vi "PCO_RecorderCreate.vi"(1 "wRecMode":u16(ring)=2 items=["PCO_RECORDER_MODE_FILE"=1, "PCO_RECORDER_MODE_MEMORY"=2, "PCO_RECORDER_MODE_CAMRAM"=3], 5 "phCamArr":u64[](array[numeric])=array[4097 elements], 7 "dwImgDistributionArr":u32[](array[numeric]), 9 "szDrive":path, 11 "error in (no error)":errorcluster {"code" format="%x"}, 12 "wFlags":u16 format="%04x") -> (4 "phRec out":u64, 6 "ErrorMessage":i32 format="%x", 8 "dwMaxImgCountArr":u32[](array[numeric]), 15 "error out":errorcluster {"code" format="%x"})   [LabVIEW 2019, in "Recorder.lvlib"]
doc: "<b>Description:</b>\nThis function creates the one and only instance of the recorder. It takes an array of handles to the required cameras as input parameter. If the function succeeds, those handles may not be used outside of the recorder until PCO_RecorderDelete is called. The main task of this function is to calculate the maximum recordable number of images for every camera by checking the available memory (RAM or Disk depending on the recorder mode) and the required distribution of the memory to the single cameras (e.g camera 1 should get twice as much available memory as camera 2, than the distribution would be [2, 1]). If the recorder is used in record to file mode, also the drive and the file type have to be specified, otherwise those parameters are just ignored.\nFunction will be rejected with error if a recorder was already created.\n\n<b>Note: </b>For file mode this function returns a warning, if the file name of the specified path already exists.\nThe function will be rejected with error if a recorder was already created.\n\n<b>Supported camera type:</b>\nAll cameras"
uses:
  Recorder.lvlib
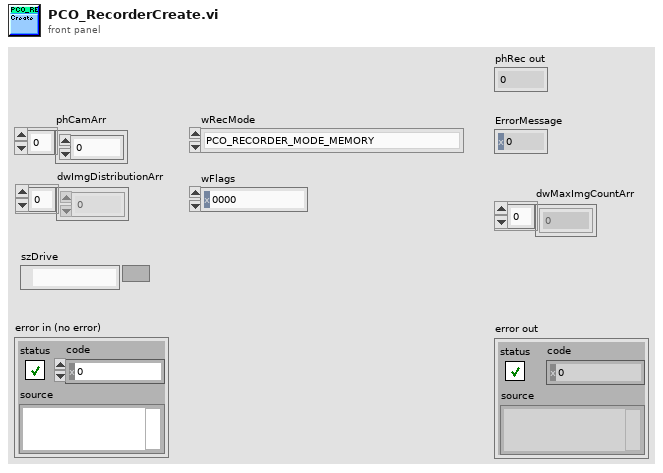
[diagram p1: front panel]
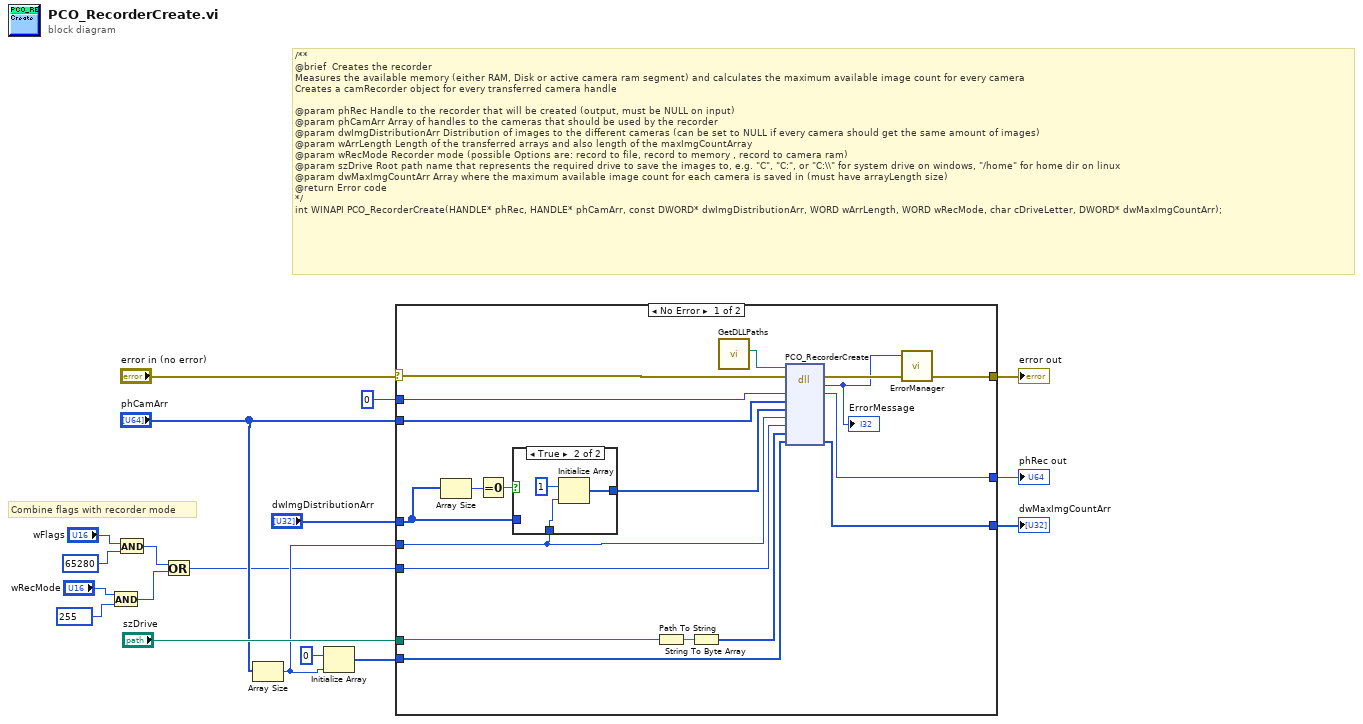
[diagram p0: block diagram]
diagram:
  # "Combine flags with recorder mode"
  # "/**\n@brief \tCreates the recorder\nMeasures the available memory (either RAM, Disk or active camera ram segment) and calculates the maximum available image count for every camera\nCreates a camRecorder object for every transferred camera handle\n\n@param phRec Handle to the recorder that will be created (output, must be NULL on input)\n@param phCamArr Array of handles to the cameras that should be used by the recorder\n@param dwImgDistributionArr Distribution of images to the different cameras (can be set to NULL if every camera should get the same amount of images)\n@param wArrLength Length of the transferred arrays and also length of the maxImgCountArray\n@param wRecMode Recorder mode (possible Options are: record to file, record to memory , record to camera ram)\n@param szDrive Root path name that represents the required drive to save the images to, e.g. \"C\", \"C:\", or \"C:\\\\\" for system drive on windows, \"/home\" for home dir on linux\n@param dwMaxImgCountArr Array where the maximum available image count for each camera is saved in (must have arrayLength size)\n@return Error code\n*/\nint WINAPI PCO_RecorderCreate(HANDLE* phRec, HANDLE* phCamArr, const DWORD* dwImgDistributionArr, WORD wArrLength, WORD wRecMode, char cDriveLetter, DWORD* dwMaxImgCountArr);"
  n1 = And(x="wRecMode", y=u16 255) -> (x .and. y?=w2:u16)
  n2 = And(x="wFlags", y=u16 65280) -> (x .and. y?=w3:u16)
  n3 = Or(x=w3, y=w2) -> (x .or. y?=w1:u16)
  n4 = Array Size(array="phCamArr") -> (size(s)=w11:i32)
  n5 = Initialize Array(u32 0 ("element"), w11) -> (w12:u32[])
  n6 = case shown="No Error" "error in (no error)" {
    selector: "error in (no error)" -> [w32 w44]
    tunnel: u64 0 ("phRec") -> [w37 w43]
    tunnel: [w36 w43] -> w18
    tunnel: "phCamArr" -> [w29 _]
    tunnel: "dwImgDistributionArr" -> [w21 _]
    tunnel: w1 -> [w35 _]
    tunnel: [w34 w42] -> w17
    tunnel: [w31 w44] -> w16
    tunnel: "szDrive" -> [w33 _]
    tunnel: w12 -> [w30 w42]
    tunnel: w11 -> [w20 _]
    frame No Error {
      n7 = Array Size(array=w21) -> (size(s)=w23:i32)
      n8 = Equal To 0?(x=w23) -> (x = 0?=w22:bool)
      n9 = case shown="True" w22 {
        tunnel: w21 -> [w38 _]
        tunnel: w20 -> [_ w40]
        tunnel: [w38 w39] -> w19
        frame False {
        }
        frame True {
          n10 = Initialize Array(u32 1 ("element"), w40) -> (w39:u32[])
        }
      }
      n11 = Path To String(path=w33) -> (string=w28:string)
      n12 = String To Byte Array(string=w28) -> (unsigned byte array=w24:u8[])
      n13 = call "GetDLLPaths.vi"() -> ("PCO_Recorder_Path"=w25:path)  [unwired: 8 in, 3 out]
      n14 = dll-call lib="?" fn="PCO_RecorderCreate"(path in=w25, error in=w32, "phRec"=w37, "phCamArr"=w29, "dwImgDistributionArr"=w19, "wArrLength"=w20, "wRecMode"=w35, "szDrive"=w24, "dwMaxImgCountArr"=w30) -> (error out=w27:errorcluster, "return type"=w26:i32, "phRec"=w36:u64, "dwMaxImgCountArr"=w34:u32[])  [unwired: 6 in, 1 out]
      "ErrorMessage" <- w26
      n15 = call "ErrorManager.vi"("error in (no error)"=w27, "error code"=w26) -> ("error out"=w31:errorcluster)  [unwired: 2 in, 1 out]
    }
    frame Error {
    }
  }
  "phRec out" <- w18
  "dwMaxImgCountArr" <- w17
  "error out" <- w16
